vi "Init.vi"() -> (1 "Max Speed":dbl, 2 "Max Power":dbl, 3 "Bed Size":cluster{"X":dbl, "Y":dbl})   [LabVIEW 2014]
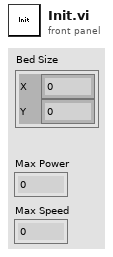
[diagram p1: front panel]
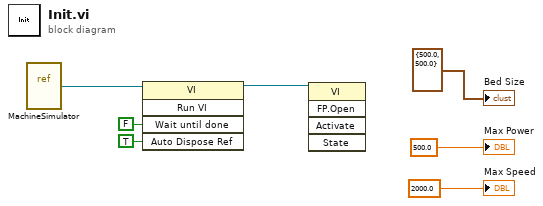
[diagram p0: block diagram]
diagram:
  n1 = vi-ref "MachineSimulator.vi"() -> (w7:refnum<vi>)
  n2 = invoke class="VI" method="Run VI"(reference=w7, "Wait until done"=FALSE ("Wait Until Done"), "Auto Dispose Ref"=TRUE ("Auto Dispose Reference")) -> (reference out=w4:refnum<vi>)  [unwired: 2 in, 4 out]
  n3 = invoke class="VI" method="FP.Open"(reference=w4) -> ()  [unwired: 4 in, 5 out]
  "Bed Size" <- cluster{"X":dbl, "Y":dbl} {"X"=500.0, "Y"=500.0} ("Bed Size")
  "Max Power" <- 500.0 ("Max Power")
  "Max Speed" <- 2000.0 ("Max Speed")
